vi "CPC_Logger.vi"(8 "error in (no error)":errorcluster) -> (0 "error out":errorcluster={"status"=TRUE, "code"=-1073807338, "source"="VISA Close in O3 ThermoScientific 49.vi"})   [LabVIEW 2013]
doc: "Use this template to build a VI to use as a subVI."
panel:
  in  "Emulation":bool
  in  "Serial Port Number":refnum<visa-resource-name>="COM3"
  in  "Save to File":bool=TRUE
  in  "file path":path=path "C:/Users/DMA2011/Desktop/o3Conc.txt"
  in  "stop":bool
  out "Waveform Chart":waveform(dbl)(graph)
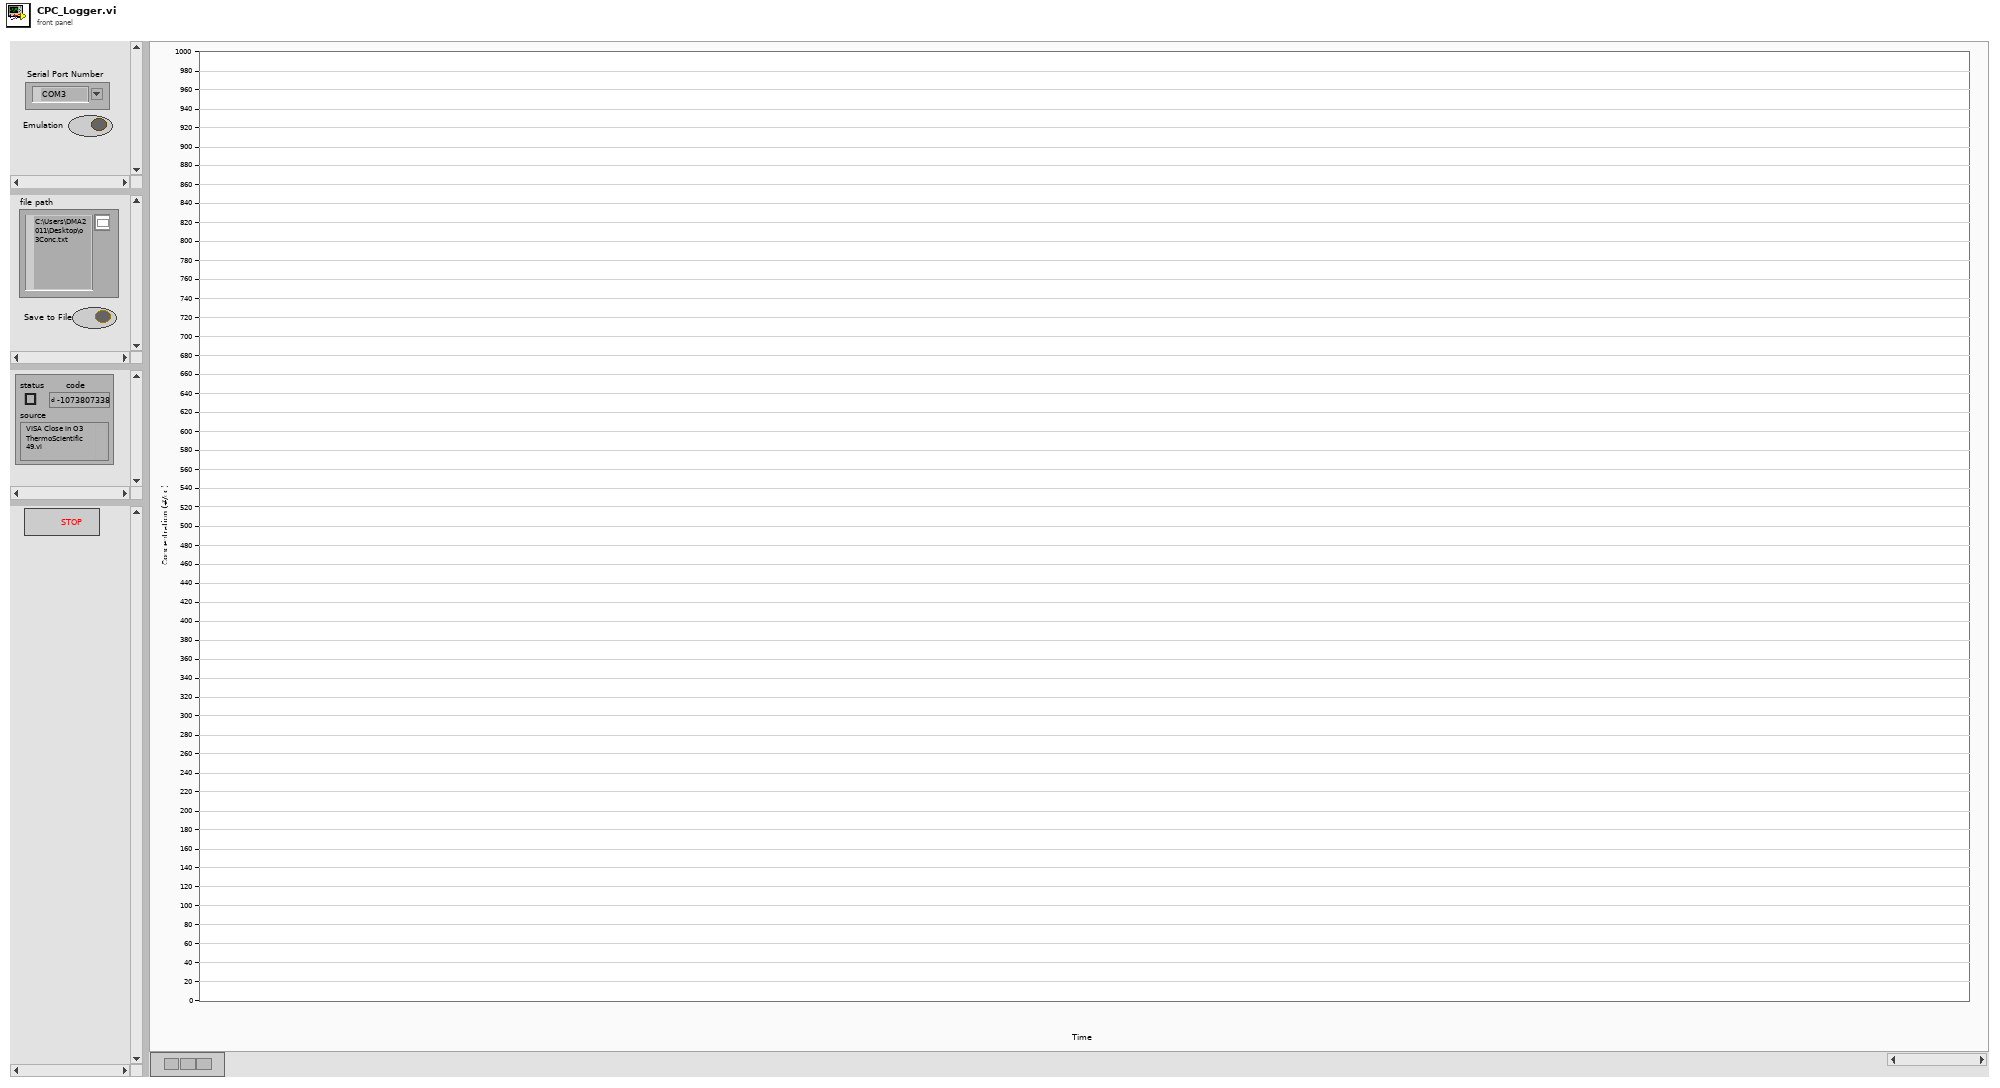
[diagram p1: front panel]
types:
  T1 = enum16{"open", "replace", "create", "open or create", "replace or create", "replace or create with confirmation"}
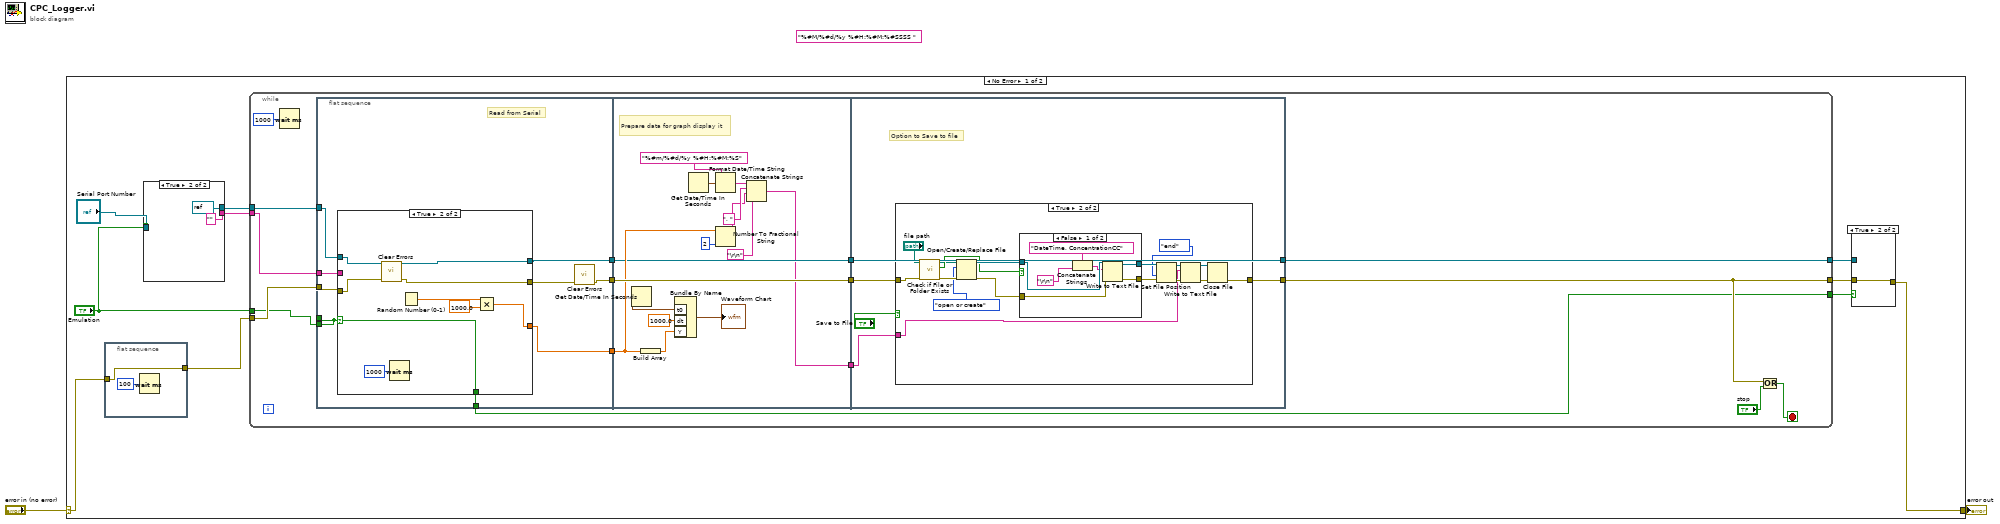
[diagram p0: block diagram]
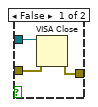
[diagram p2: hidden frame]
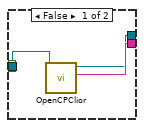
[diagram p3: hidden frame]
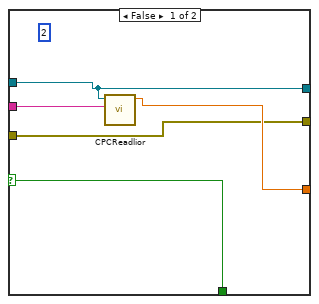
[diagram p4: hidden frame]
diagram:
  (unwired) "%#M/%#d/%y %#H:%#M:%#SSSS " ("string")
  n1 = case shown="No Error" "error in (no error)" {
    selector: "error in (no error)" -> [w6 w109]
    tunnel: [w10 w109] -> w1
    frame No Error {
      n2 = flat-sequence {
        tunnel: w6 -> [w22]
        tunnel: [w22] -> w5
        frame #0 {
          n3 = Wait (ms)(milliseconds to wait=u32 100) -> ()  [unwired: 1 out]
        }
      }
      n4 = case shown="True" "Emulation" {
        tunnel: "Serial Port Number" -> [w19 _]
        tunnel: [w18 "" ("CPC model")] -> w8
        tunnel: [w17 refnum<visa-resource-name> refnum ("dup CPC port")] -> w7
        frame False {
          n5 = call "OpenCPClior.vi"("CPC port"=w19) -> ("CPC model"=w18:string, "dup CPC port"=w17:refnum<visa-resource-name>)  [unwired: 8 in, 1 out]
        }
        frame True {
        }
      }
      n6 = while {
        tunnel: w5 -> [w35]
        tunnel: [w37] -> w12
        tunnel: [w39] -> w11
        tunnel: w8 -> [w29]
        tunnel: w7 -> [w28]
        tunnel: "Emulation" -> [w25]
        tunnel: [w24] -> w3
        stop <- w36 stop-if-true
        n7 = Wait (ms)(milliseconds to wait=u32 1000) -> ()  [unwired: 1 out]
        n8 = flat-sequence {
          tunnel: [w41] -> _
          tunnel: w35 -> [w48]
          tunnel: [w46] -> w30
          tunnel: w29 -> [w45]
          tunnel: w28 -> [w44]
          tunnel: [w43] -> w27
          tunnel: [w42] -> w26
          tunnel: w25 -> [w41]
          tunnel: [w40] -> w24
          tunnel: [w63] -> w34
          tunnel: [w72] -> w33
          tunnel: [w62] -> w32
          tunnel: w30 -> [w72]
          tunnel: w27 -> [w64]
          tunnel: w26 -> [w63]
          tunnel: [w77] -> w37
          tunnel: [w81] -> w39
          tunnel: w34 -> [w81]
          tunnel: w33 -> [w78]
          tunnel: w32 -> [w79]
          frame #0 {
            # "Read from Serial"
            n9 = case shown="True" w41 {
              selector: w41 -> [w49 w57]
              tunnel: [w50 w59] -> w47
              tunnel: w48 -> [w50 w60]
              tunnel: w45 -> [w52 _]
              tunnel: w44 -> [w51 w58]
              tunnel: [w53 w54] -> w43
              tunnel: [w51 w58] -> w42
              tunnel: [w49 w57] -> w40
              frame False {
                (unwired) 2
                n10 = call "CPCReadlior.vi"("model"=w52, "CPC port"=w51) -> ("concentration part/cm3"=w53:dbl)  [unwired: 8 in, 1 out]
              }
              frame True {
                n11 = call <vilib>:"Clear Errors.vi"("error in (no error)"=w60) -> ("error out"=w59:errorcluster)  [unwired: 6 in]
                n12 = Wait (ms)(milliseconds to wait=u32 1000) -> ()  [unwired: 1 out]
                n13 = Random Number (0-1)() -> (number: 0 to 1=w56:dbl)
                n14 = Multiply(x=w56, y=1000.0) -> (x*y=w54:dbl)
              }
            }
            n15 = call <vilib>:"Clear Errors.vi"("error in (no error)"=w47) -> ("error out"=w46:errorcluster)  [unwired: 6 in]
          }
          frame #1 {
            # "Prepare data for graph display it"
            n16 = Get Date/Time In Seconds() -> (seconds since 1Jan1904=w76:timestamp)
            n17 = Build Array(w64) -> (w74:dbl[])
            n18 = Bundle By Name("t0"=w76, "dt"=1000.0, "Y"=w74) -> (→"Waveform Chart":waveform(dbl))  [unwired: 1 in]
            n19 = Get Date/Time In Seconds() -> (seconds since 1Jan1904=w71:timestamp)
            n20 = Format Date/Time String(time format string (%c)="%#m/%#d/%y %#H:%#M:%S" ("string"), seconds (now)=w71) -> (date/time string=w70:string)  [unwired: 1 in]
            n21 = Number To Fractional String(number=w64, precision (6)=i16 2) -> (F-format string=w65:string)  [unwired: 2 in]
            n22 = Concatenate Strings(w70, ", " ("string"), w65, "\r\n") -> (w62:string)
          }
          frame #2 {
            # "Option to Save to file"
            n23 = case shown="True" "Save to File" {
              tunnel: w79 -> [_ w83]
              tunnel: w78 -> [w82 w86]
              tunnel: [w82 w85] -> w77
              frame False {
              }
              frame True {
                n24 = call <vilib>:"Check if File or Folder Exists.vi"("error in (no error)"=w86, "path"="file path") -> ("error out"=w88:errorcluster, "file or folder exists?"=w90:bool, "dup path"=w89:path)  [unwired: 7 in]
                n25 = Open/Create/Replace File(file path (use dialog)=w89, error in=w88, operation (0:open)=T1."open or create") -> (refnum out=w91:refnum<file>, error out=w92:errorcluster)  [unwired: 3 in, 1 out]
                n26 = case shown="False" w90 {
                  tunnel: w91 -> [w105 w108]
                  tunnel: w92 -> [w103 w107]
                  tunnel: [w102 w107] -> w96
                  tunnel: [w101 w108] -> w98
                  frame False {
                    n27 = Concatenate Strings("DateTime, ConcentrationCC" ("string"), "\r\n") -> (w104:string)
                    n28 = Write to Text File(file (use dialog)=w105, text=w104, error in=w103) -> (refnum out=w101:refnum<file>, error out=w102:errorcluster)  [unwired: 1 in, 1 out]
                  }
                  frame True {
                  }
                }
                n29 = Set File Position(refnum=w98, from (0:start)=enum16{"start", "end", "current"}."end", error in=w96) -> (refnum out=w99:refnum<file>, error out=w97:errorcluster)  [unwired: 1 in]
                n30 = Write to Text File(file (use dialog)=w99, text=w83, error in=w97) -> (refnum out=w93:refnum<file>, error out=w94:errorcluster)  [unwired: 1 in, 1 out]
                n31 = Close File(refnum=w93, error in=w94) -> (error out=w85:errorcluster)  [unwired: 1 out]
              }
            }
          }
        }
        n32 = Or(x=w37, y="stop") -> (x .or. y?=w36:bool)
      }
      n33 = case shown="True" w3 {
        tunnel: w12 -> [w15 w16]
        tunnel: w11 -> [w14 _]
        tunnel: [w13 w16] -> w10
        frame False {
          n34 = VISA Close(VISA resource name=w14, error in (no error)=w15) -> (error out=w13:errorcluster)
        }
        frame True {
        }
      }
    }
    frame Error {
    }
  }
  "error out" <- w1
